vi "FTW-Ether-Address-Build.vi"(5 "Path":string, 7 "Message Transport Scheme":T1, 11 "error in":errorcluster) -> (6 "Endpoint Address":string, 15 "error out":errorcluster)   [LabVIEW 2013, in "FTW-Actor.lvlib" / "FTW-Ether.lvclass"]
uses:
  FTW-Ether.lvclass
  FTW-Ether-MessageTransportScheme.ctl
panel:
  # "Inputs"
  # "Outputs"
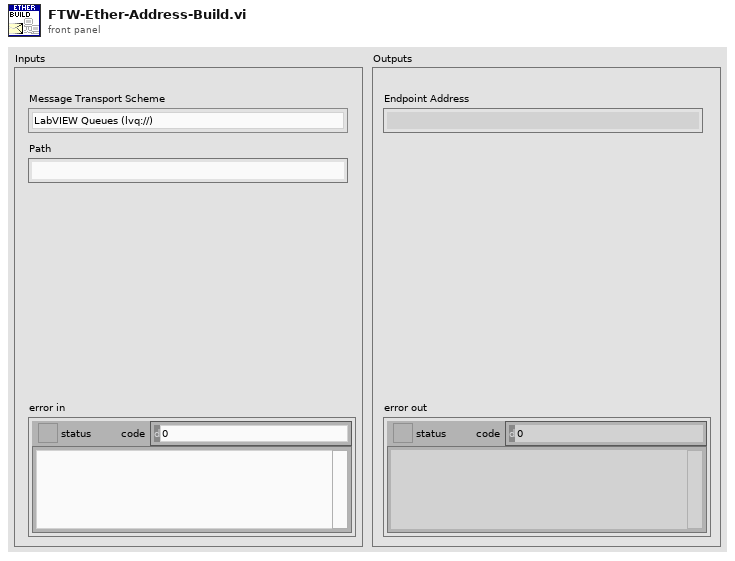
[diagram p1: front panel]
types:
  T1 = typedef "FTW-Actor.lvlib/FTW-Ether.lvclass/FTW-Ether-MessageTransportScheme.ctl" = enum16{"LabVIEW Queues (lvq://)", "LabVIEW Notifiers (lvn://)", "LabVIEW Network Streams (lvns://)"}
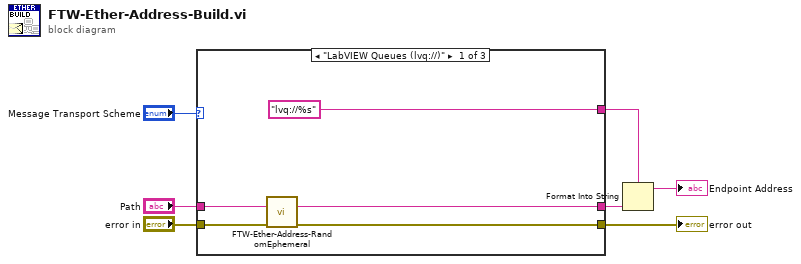
[diagram p0: block diagram]
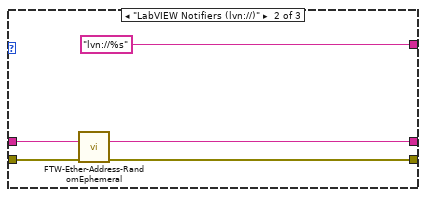
[diagram p2: hidden frame]
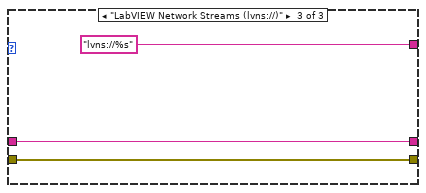
[diagram p3: hidden frame]
diagram:
  n1 = case shown="\"LabVIEW Queues (lvq://)\"" "Message Transport Scheme" {
    tunnel: ["lvq://%s" ("format string") "lvn://%s" ("format string") "lvns://%s" ("format string")] -> w6
    tunnel: "Path" -> [w11 w16 w19]
    tunnel: [w8 w13 w19] -> w3
    tunnel: "error in" -> [w10 w15 w18]
    tunnel: [w9 w14 w18] -> w1
    frame "LabVIEW Queues (lvq://)" {
      n2 = call "FTW-Ether-Address-RandomEphemeral.vi"("Endpoint"=w11, "error in"=w10) -> ("Endpoint with Replacements"=w8:string, "error out"=w9:errorcluster)  [unwired: 12 in]
    }
    frame "LabVIEW Notifiers (lvn://)" {
      n3 = call "FTW-Ether-Address-RandomEphemeral.vi"("Endpoint"=w16, "error in"=w15) -> ("Endpoint with Replacements"=w13:string, "error out"=w14:errorcluster)  [unwired: 12 in]
    }
    frame "LabVIEW Network Streams (lvns://)" {
    }
  }
  "error out" <- w1
  n4 = Format Into String(format string=w6, w3) -> (resulting string=→"Endpoint Address":string)  [unwired: 2 in, 1 out]
